vi "Write Formatter.vi"(8 "error in (no error)":errorcluster, 10 "Formatter":refnum<k38>, 11 "Formatter in":refnum<class "Formatter.lvclass">) -> (0 "error out":errorcluster, 3 "Formatter out":refnum<class "Formatter.lvclass">)   [LabVIEW 2022 SP3, in "Logger.lvlib" / "Formatter.lvclass"]
uses:
  Formatter.lvclass
  Formatter.lvclass/Formatter.ctl
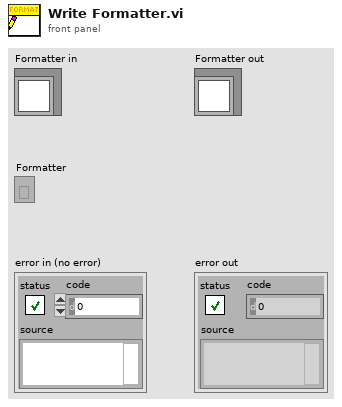
[diagram p1: front panel]
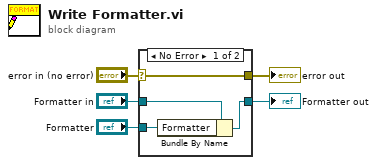
[diagram p0: block diagram]
diagram:
  n1 = case shown="No Error" "error in (no error)" {
    selector: "error in (no error)" -> [w9 w10]
    tunnel: [w9 w10] -> w4
    tunnel: [w7 w11] -> w2
    tunnel: "Formatter in" -> [w8 w11]
    tunnel: "Formatter" -> [w6 _]
    frame No Error {
      n2 = Bundle By Name(cluster=w8, "Formatter"=w6) -> (w7:refnum<class "Formatter.lvclass">)
    }
    frame Error {
    }
  }
  "error out" <- w4
  "Formatter out" <- w2
